vi "Finish Move.vi"(8 "error in (no error)":errorcluster, 11 "SwipeMenu in":refnum<class "SwipeMenu.lvclass">) -> (0 "error out":errorcluster, 3 "SwipeMenu out":refnum<class "SwipeMenu.lvclass">)   [LabVIEW 2019, in "SwipeMenu.lvclass"]
uses:
  SwipeMenu.lvclass
  SwipeMenu.lvclass/SwipeMenu.ctl
  <vilib>/Utility/inputDevices.llb/mouseAcquire.vi
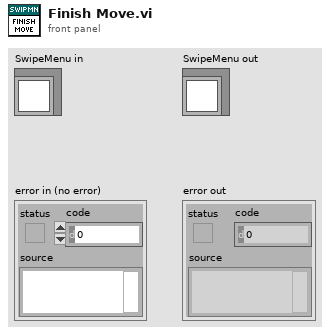
[diagram p1: front panel]
types:
  T1 = cluster{"Horizontal":i32, "Vertical":i32, "Scrolling":i32}
  T2 = typedef "LVPointTypeDef.ctl" = cluster{"Horizontal":i16, "Vertical":i16}
  T3 = enum16{"Idle", "Mouse Nav", "Slowdown", "Button Nav"}
  T4 = typedef "SwipeMenu.lvclass/State Data.ctl" = cluster{"State":enum16{"Idle", "Mouse Nav", "Slowdown", "Button Nav"}, "Timeout":i32, "Time":timestamp, "Position":i32, "Scroll Position":i16, "Rate":dbl, "Direction":enum16{"Left", "Right"}}
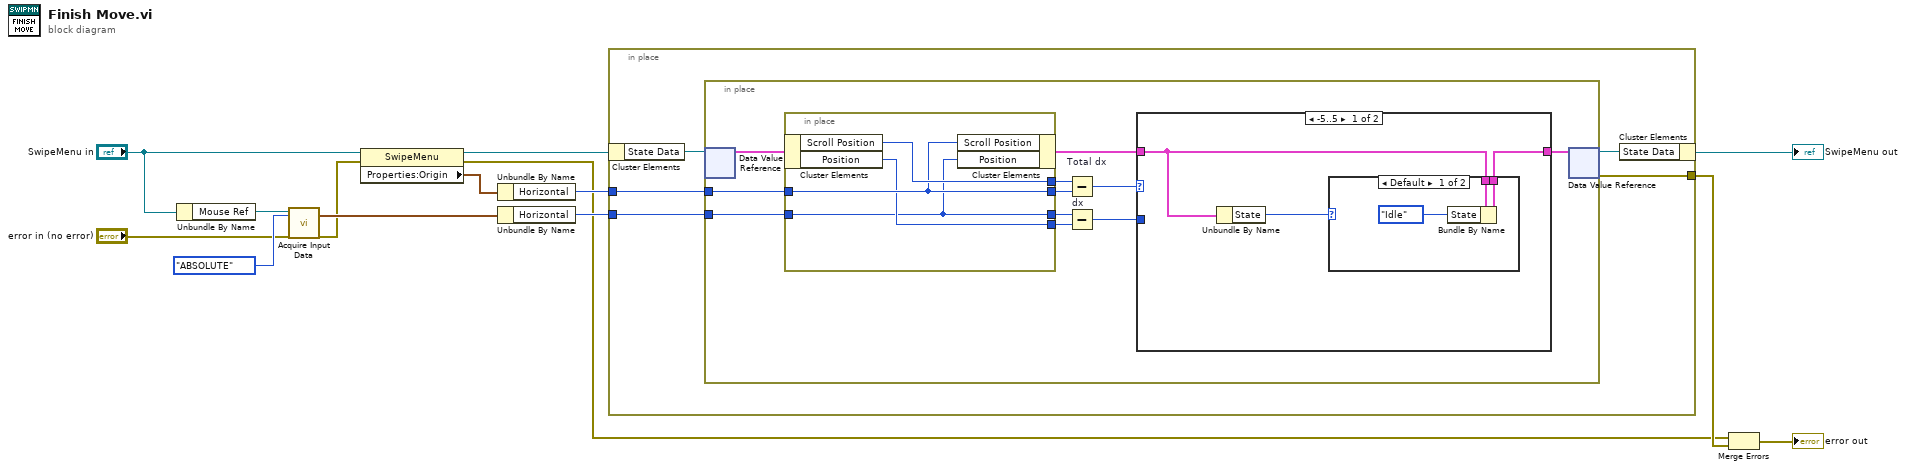
[diagram p0: block diagram]
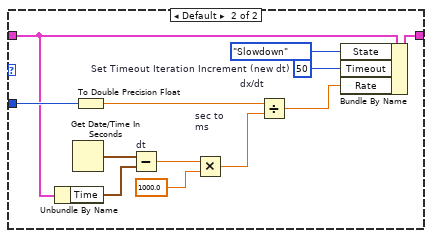
[diagram p3: hidden frame]
diagram:
  n1 = Unbundle By Name("SwipeMenu in") -> ("Mouse Ref"=w14:refnum<k1>)
  n2 = call-poly <vilib>:"Acquire Input Data.vi"("device ID"=w14, "key mode"=enum16{"RELATIVE", "ABSOLUTE"}."ABSOLUTE", "error in (no error)"="error in (no error)") -> ("axis info"=w13:T1, "error out"=w10:errorcluster)  [unwired: 13 in, 2 out]
  n3 = property on="Property Node" class="SwipeMenu"(reference="SwipeMenu in", error in=w10) -> (reference out=w9:refnum<class "SwipeMenu.lvclass">, error out=w3:errorcluster, "Properties:Origin"=w7:T2)
  n4 = Unbundle By Name(w7) -> ("Horizontal"=w6:i16)
  n5 = Unbundle By Name(w13) -> ("Horizontal"=w8:i32)
  n6 = in-place {
    in-place-border: w8 -> [w18]
    in-place-border: w6 -> [w17]
    in-place-border: [w15] -> w4
    n7 = in-place-cluster #1(w9) -> ("State Data"=w19:refnum<data-value>)
    n8 = in-place {
      in-place-border: w18 -> [w22]
      in-place-border: w17 -> [w30]
      n9 = in-place-dvr #2(w19) -> (w23:T4)  [unwired: 1 out]
      n10 = in-place {
        in-place-border: [w34] -> w26
        in-place-border: w30 -> [w33]
        in-place-border: [w33] -> w25
        in-place-border: w22 -> [w31]
        in-place-border: [w32] -> w21
        in-place-border: [w31] -> w20
        n11 = in-place-cluster #3(w23) -> ("Scroll Position"=w34:i16, "Position"=w32:i32)
        n12 = in-place-cluster #3("Scroll Position"=w33, "Position"=w31) -> (w28:T4)
      }
      n13 = Subtract "Total dx"(x=w26, y=w25) -> (x-y=w24:i16)
      n14 = Subtract "dx"(x=w20, y=w21) -> (x-y=w29:i32)
      n15 = case shown="-5..5" w24 {
        tunnel: w28 -> [w36 w44]
        tunnel: [w37 w43] -> w27
        tunnel: w29 -> [_ w49]
        frame -5..5 {
          n16 = Unbundle By Name(w36) -> ("State"=w35:T3)
          n17 = case shown="Default" w35 {
            tunnel: [w40 w41] -> w37
            tunnel: w36 -> [w39 w41]
            frame Default {
              n18 = Bundle By Name(cluster=w39, "State"=T3."Idle") -> (w40:T4)
            }
            frame "Slowdown" {
            }
          }
        }
        frame Default {
          w46 = 50  # Set Timeout Iteration Increment (new dt)
          n19 = Unbundle By Name(w44) -> ("Time"=w51:timestamp)
          n20 = Get Date/Time In Seconds() -> (seconds since 1Jan1904=w52:timestamp)
          n21 = To Double Precision Float(number=w49) -> (double precision float=w48:dbl)
          n22 = Subtract "dt"(x=w52, y=w51) -> (x-y=w53:dbl)
          n23 = Multiply "sec to\nms"(x=w53, y=1000.0) -> (x*y=w47:dbl)
          n24 = Divide "dx/dt"(x=w48, y=w47) -> (x/y=w45:dbl)
          n25 = Bundle By Name(cluster=w44, "State"=T3."Slowdown", "Timeout"=w46, "Rate"=w45) -> (w43:T4)
        }
      }
      n26 = in-place-dvr #2(w27) -> (w16:refnum<data-value>, w15:errorcluster)
    }
    n27 = in-place-cluster #1("State Data"=w16) -> (→"SwipeMenu out":refnum<class "SwipeMenu.lvclass">)
  }
  n28 = Merge Errors(w3, w4) -> (→"error out":errorcluster)
